vi "update_volume.vi"(1 "Volume In":dbl, 2 "Action":u8(ring) items=["add to volume", "set volume "]) -> (0 "Current Volume":dbl)   [LabVIEW 2010]
doc: "This VI takes care of update access to the HCl volume global. Reading from the global can still be done directly, but using this VI will ensure that updates to the HCl data are handled sequentially and don't overwrite eachother (race condition). If later developers find themselves making the flow of volume information around the application more complicated, it would be worth modifying this vi to behave more like an action action (possibly removing the global entirely). For now though, the flow is simple enough that a global is fine, but again, continuing to use this VI for updates will add to the consitence and ease up later upgradability of the application."
uses:
  HCl_volume_global.vi
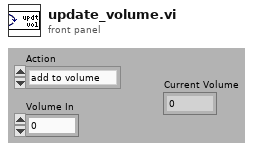
[diagram p1: front panel]
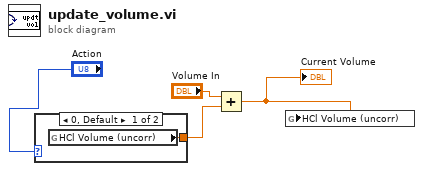
[diagram p0: block diagram]
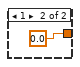
[diagram p2: hidden frame]
diagram:
  n1 = case shown="0, Default" "Action" {
    tunnel: [w5 0.0] -> w4
    frame 0, Default {
      n2 = global read "HCl_volume_global.vi" "HCl Volume (uncorr)"() -> (w5:dbl)
    }
    frame 1 {
    }
  }
  n3 = Add(x="Volume In", y=w4) -> (x+y=w2:dbl)
  "Current Volume" <- w2
  n4 = global write "HCl_volume_global.vi" "HCl Volume (uncorr)"(w2) -> ()
